vi "testThreshold.vi"() -> ()   [LabVIEW 2009]
uses:
  <vilib>/Utility/NIReport.llb/NI_report.lvclass
  <vilib>/Utility/NIReport.llb/HTML/NI_HTML.lvclass
panel:
  in  "Channel":i8
  in  "Treshold":i16(slide) min=0 max=1000 scale=0.0..1000.0
  in  "stop":bool
  out "error out":errorcluster
  in  "Instrument VISA in":T1={"AWG VISA"="generadorpulsos", "Oscilloscope  VISA "="Oscilloscope", "Integration Board IP"="172.16.7.43", "connection ID"=refnum, "report out"=refnum, "report file path"=path "C:/Documents and Settings/CTA_LAB01/Desktop/L0_Asic/L0 Asic Test Data"}
  in  "error in":errorcluster
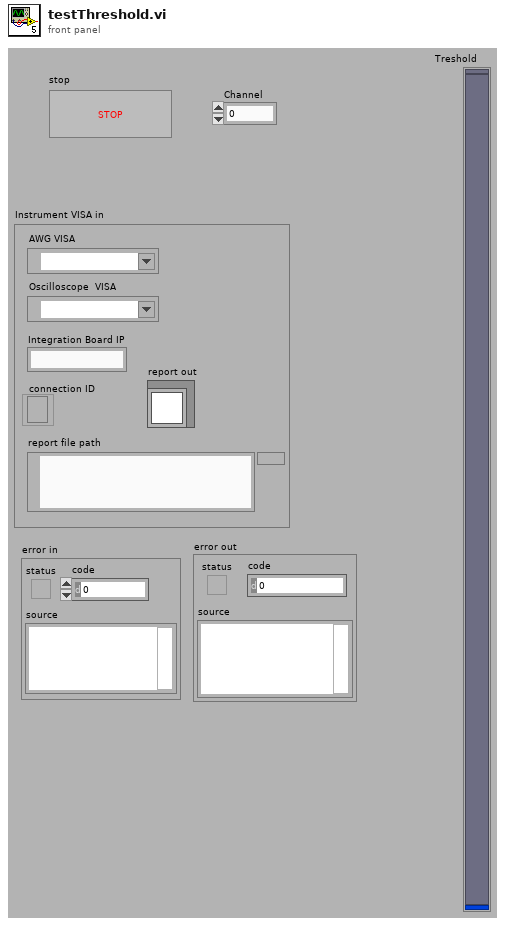
[diagram p1: front panel]
types:
  T1 = cluster{"AWG VISA":refnum<visa-resource-name>, "Oscilloscope  VISA ":refnum<visa-resource-name>, "Integration Board IP":string, "connection ID":refnum<k5>, "report out":refnum<class "NI_report.lvclass">, "report file path":path}
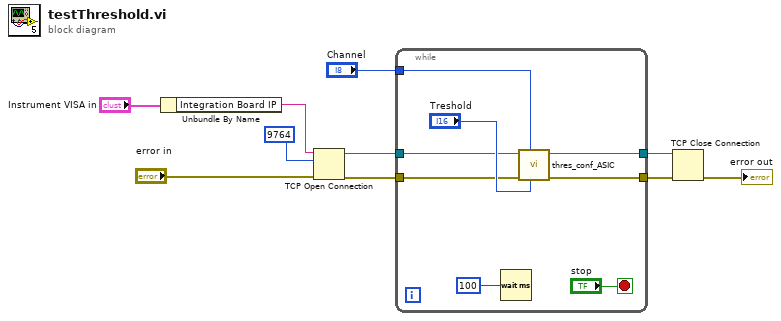
[diagram p0: block diagram]
diagram:
  n1 = Unbundle By Name("Instrument VISA in") -> ("Integration Board IP"=w8:string)
  n2 = TCP Open Connection(address=w8, remote port or service name=u16 9764, error in (no error)="error in") -> (connection ID=w4:refnum<k5>, error out=w5:errorcluster)  [unwired: 2 in]
  n3 = while {
    tunnel: w5 -> [w16]
    tunnel: w4 -> [w15]
    tunnel: "Channel" -> [w13]
    tunnel: [w12] -> w2
    tunnel: [w11] -> w1
    stop <- "stop" stop-if-true
    n4 = Wait (ms)(milliseconds to wait=u32 100 ("Ib_clipVb")) -> ()  [unwired: 1 out]
    n5 = call "thres_conf_ASIC.vi"("threshold"="Treshold", "Ring"=w13, "error out 3"=w16, "connection ID"=w15) -> ("error out 2"=w11:errorcluster, "connection ID out"=w12:refnum<k5>)  [unwired: 4 in, 2 out]
  }
  n6 = TCP Close Connection(connection ID=w2, error in (no error)=w1) -> (error out=→"error out":errorcluster)  [unwired: 1 in, 1 out]
